vi "1D Array to String_csm.vi"(7 "delimiter (Tab)":string, 10 "Array of Strings":string[](array[string])) -> (1 "delimited string":string)   [LabVIEW 2017, in "API String Arguments Support.lvlib"]
doc: "Converts 1D Array of strings to a delimited string"
uses:
  API String Arguments Support.lvlib
panel:
  # "[OpenG VI Tags] ***Do Not Remove***"
  # "1D Array to String.vi\n\nConverts 1D Array of strings to a delimited string.\n\nPlease visit http://www.OpenG.org to learn about the\nOpen Source LabVIEW software movement.\n\nNOTICE -- YOU MUST LEAVE THIS NOTICE IN PLACE.  PER THE TERMS OF THE LICENSE BELOW, YOU MAY SUBLICENSE THIS SOFTWARE \nIN ANY WAY THAT DOES NOT CONFLICT WITH THIS LICENSE.\n\n### BSD License (http://www.opensource.org/licenses/bsd-license.php) Begin ###\n \nCopyright (c) 2002, Jim Kring <jim@jimkring.com>\n\nAll rights reserved.\n\nRedistribution and use in source and binary forms, with or without modification, are permitted provided that the following conditions are met:\n\n    * Redistributions of source code must retain the above copyright notice, this list of conditions and the following disclaimer.\n    * Redistributions in binary form must reproduce the above copyright notice, this list of conditions and the following disclaimer in the \n       documentation and/or other materials provided with the distribution.\n    * Neither the name of SciWare, James Kring, Inc., nor the names of its contributors may be used to endorse or promote products derived \n       from this software without specific prior written permission.\n\nTHIS SOFTWARE IS PROVIDED BY THE COPYRIGHT HOLDERS AND CONTRIBUTORS \"AS IS\" AND ANY EXPRESS OR IMPLIED WARRANTIES, \nINCLUDING, BUT NOT LIMITED TO, THE IMPLIED WARRANTIES OF MERCHANTABILITY AND FITNESS FOR A PARTICULAR PURPOSE ARE \nDISCLAIMED. IN NO EVENT SHALL THE COPYRIGHT OWNER OR CONTRIBUTORS BE LIABLE FOR ANY DIRECT, INDIRECT, INCIDENTAL,\n SPECIAL, EXEMPLARY, OR CONSEQUENTIAL DAMAGES (INCLUDING, BUT NOT LIMITED TO, PROCUREMENT OF SUBSTITUTE GOODS OR \nSERVICES; LOSS OF USE, DATA, OR PROFITS; OR BUSINESS INTERRUPTION) HOWEVER CAUSED AND ON ANY THEORY OF LIABILITY, \nWHETHER IN CONTRACT, STRICT LIABILITY, OR TORT (INCLUDING NEGLIGENCE OR OTHERWISE) ARISING IN ANY WAY OUT OF THE USE \nOF THIS SOFTWARE, EVEN IF ADVISED OF THE POSSIBILITY OF SUCH DAMAGE.\n\n### BSD License End ###"
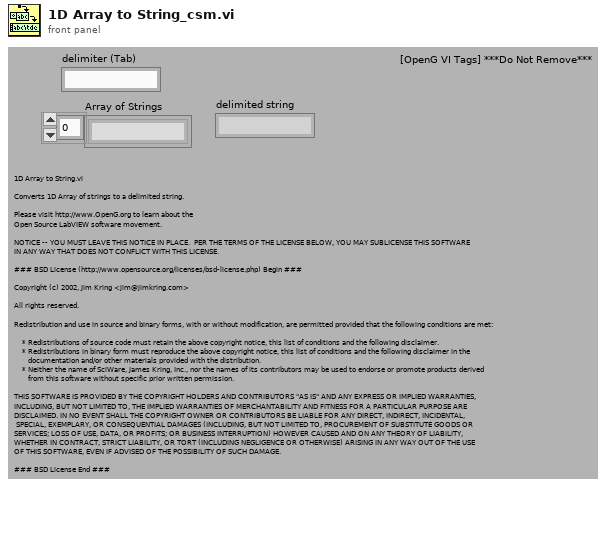
[diagram p1: front panel]
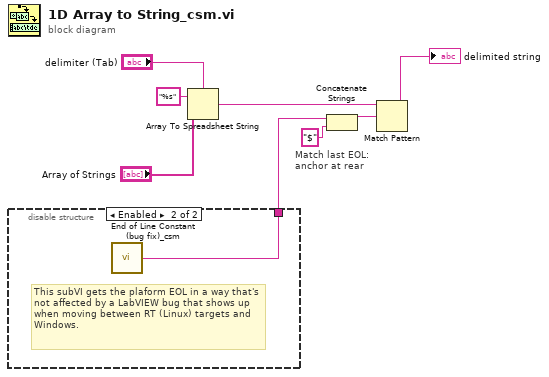
[diagram p0: block diagram]
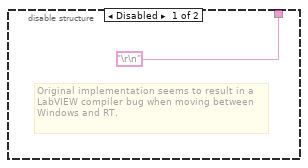
[diagram p2: hidden frame]
diagram:
  # "Match last EOL:\nanchor at rear"
  n1 = disable-structure shown="Enabled" {
    disable-tunnel: ["\r\n" w10] -> w1
    frame Disabled {
      # "Original implementation seems to result in a LabVIEW compiler bug when moving between Windows and RT."
    }
    frame Enabled {
      # "This subVI gets the plaform EOL in a way that's not affected by a LabVIEW bug that shows up when moving between RT (Linux) targets and Windows."
      n2 = call "End of Line Constant (bug fix)_csm.vi"() -> ("Platform EOL"=w10:string)  [unwired: 5 in]
    }
  }
  n3 = Array To Spreadsheet String(delimiter (Tab)="delimiter (Tab)", array="Array of Strings", 3:"%s" ("format string")) -> (spreadsheet string=w2:string)
  n4 = Concatenate Strings(w1, "$" ("Substring")) -> (w3:string)
  n5 = Match Pattern(string=w2, regular expression=w3) -> (before substring=→"delimited string":string)  [unwired: 1 in, 3 out]
